vi "Matches.vi"(8 "error in (no error)":errorcluster, 10 "Actual":variant, 11 "IsEqual in":refnum<class "IsEqual.lvclass">) -> (0 "error out":errorcluster, 2 "Result":bool, 3 "IsEqual out":refnum<class "IsEqual.lvclass">)   [LabVIEW 2017, in "Constraint.lvlib" / "IsEqual.lvclass"]
doc: "Evaluates the constraint for <B>Actual</B>. Returns true if the constraint is met."
uses:
  IsEqual.lvclass
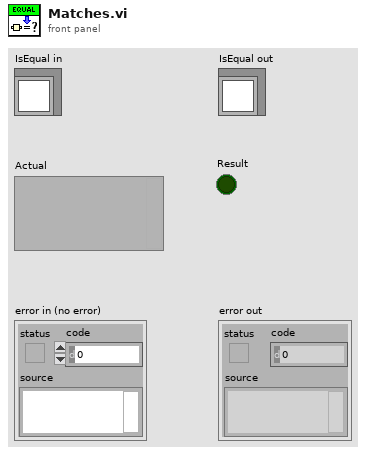
[diagram p1: front panel]
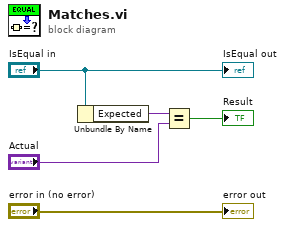
[diagram p0: block diagram]
diagram:
  n1 = Unbundle By Name("IsEqual in") -> ("Expected"=w2:variant)
  n2 = Equal?(x=w2, y="Actual") -> (x = y?=→"Result":bool)
  "error out" <- "error in (no error)"
  "IsEqual out" <- "IsEqual in"
